vi "Configure Burst.vi"(4 "Busrt Delay  (0.0s)":dbl format="%#.6g", 5 "Burst Cont":bool, 6 "Burst Count (5)":i32=5, 7 "Enable Burst (T: Enable)":bool=TRUE, 8 "error in (no error)":errorcluster, 9 "Burst Mode (0: Triggered)":u16(ring) items=["Triggered", "Gated"], 10 "Channel (0: Channel 1)":u16(ring) items=["Channel 1", "Channel 2"], 11 "VISA resource name":refnum<visa-resource-name>) -> (0 "error out":errorcluster, 3 "VISA resource name out":refnum<visa-resource-name>)   [LabVIEW 2019, in "Tektronix AFG 3000 Series.lvlib"]
doc: "Allows and configures burst modulation. Configures the function generator to output a waveform with specified number of cycles, called burst. The carrier waveform shape and parameters are set by Configure Standard Waveform."
uses:
  <userlib>/Tektronix AFG 3000 Series/Tektronix AFG 3000 Series.lvlib
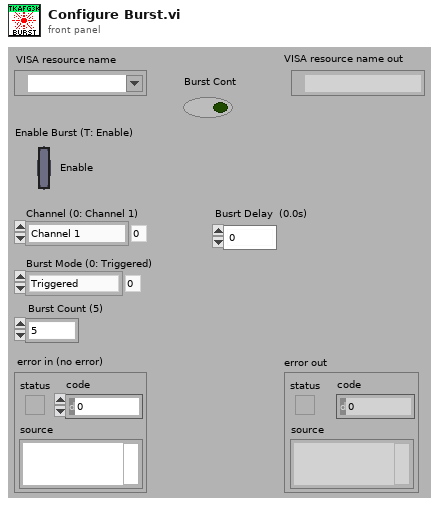
[diagram p1: front panel]
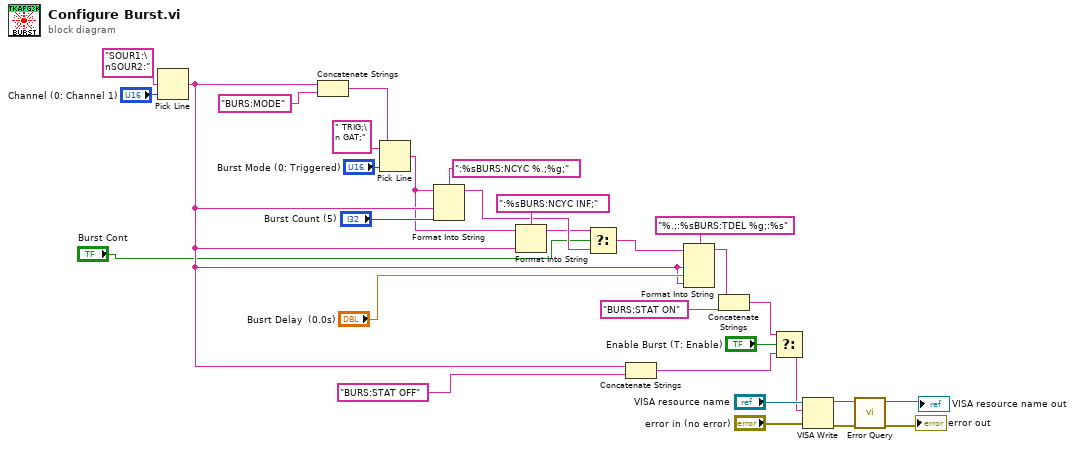
[diagram p0: block diagram]
diagram:
  n1 = Pick Line(multi-line string="SOUR1:\nSOUR2:" ("string (\"\")"), line index="Channel (0: Channel 1)") -> (output string=w6:string)  [unwired: 1 in]
  n2 = Concatenate Strings(w6, "BURS:MODE" ("format string")) -> (w13:string)
  n3 = Pick Line(string ("")=w13, multi-line string=" TRIG;\n GAT;" ("string (\"\")"), line index="Burst Mode (0: Triggered)") -> (output string=w2:string)
  n4 = Format Into String(format string=":%sBURS:NCYC %.;%g;", initial string=w2, w6, "Burst Count (5)") -> (resulting string=w5:string)  [unwired: 1 in, 1 out]
  n5 = Format Into String(format string=":%sBURS:NCYC INF;", initial string=w2, w6) -> (resulting string=w4:string)  [unwired: 1 in, 1 out]
  n6 = Select(t=w4, s="Burst Cont", f=w5) -> (s? t:f=w3:string)
  n7 = Concatenate Strings(w6, "BURS:STAT OFF" ("string")) -> (w12:string)
  n8 = Format Into String(format string="%.;:%sBURS:TDEL %g;:%s", initial string=w3, w6, "Busrt Delay  (0.0s)", w6) -> (resulting string=w8:string)  [unwired: 1 in, 1 out]
  n9 = Concatenate Strings(w8, "BURS:STAT ON" ("string")) -> (w20:string)
  n10 = Select(t=w20, s="Enable Burst (T: Enable)", f=w12) -> (s? t:f=w18:string)
  n11 = VISA Write(VISA resource name="VISA resource name", write buffer=w18, error in (no error)="error in (no error)") -> (VISA resource name out=w28:refnum<visa-resource-name>, error out=w27:errorcluster)  [unwired: 1 out]
  n12 = call <userlib>:"Error Query.vi"("error in (no error)"=w27, "VISA resource name"=w28) -> ("error out"=→"error out":errorcluster, "VISA resource name out"=→"VISA resource name out":refnum<visa-resource-name>)  [unwired: 6 in, 2 out]
